vi "NIFPGA-MCS.ProcCases.vi"(0 "i ref in":refnum<vi>, 1 "selector":string, 2 "Data":T1, 3 "call cluster":T2={"Object"="", "Selector"="", "CallType"=enum."synchronous", "Async Object"="", "Async Selector"="", "Data Descriptor"="", "Data"=[], "Error #"=0, "Expire"=0}, 5 "error in (no error)":errorcluster) -> (14 "i ref out":refnum<vi>, 17 "answer cluster":T2={"Object"="", "Selector"="", "CallType"=enum."synchronous", "Async Object"="", "Async Selector"="", "Data Descriptor"="", "Data"=[], "Error #"=0, "Expire"=0}, 19 "error out":errorcluster)   [LabVIEW 2014, in "NIFPGA-MCS.lvlib"]
doc: "This method is called by a process from within the default case in the event loop. The methods of a class that are linked to events will be called from THIS method. Add your code here."
uses:
  NIFPGA-MCS.lvlib
  CSCore/CSSystem/CoreDefs/CoreDefs.call_type.ctl
  CSCore/BaseProcess/BaseProcess.descriptor string definition.ctl
  CSCore/CSSystem/CoreDefs/CoreDefs.rawDataType.ctl
  CSCore/CSSystem/CoreLib/CoreLib.string 2 byte array.vi
  CSCore/CSSystem/CoreLib/CoreLib.short 2 byte array.vi
  CSCore/CSSystem/CoreLib/CoreLib.int 2 byte array.vi
  CSCore/CSSystem/CoreLib/CoreLib.byte array 2 int.vi
  CSCore/CSSystem/CoreLib/CoreLib.double 2 byte array.vi
  CSCore/CSSystem/CoreLib/CoreLib.byte array 2 double.vi
  CSCore/CSSystem/CoreLib/CoreLib.lvlib
  CSCore/BaseProcess/BaseProcess.lvlib
  CSCore/CSApplicationBaseClasses/MCSBase/MCSBase.lvlib
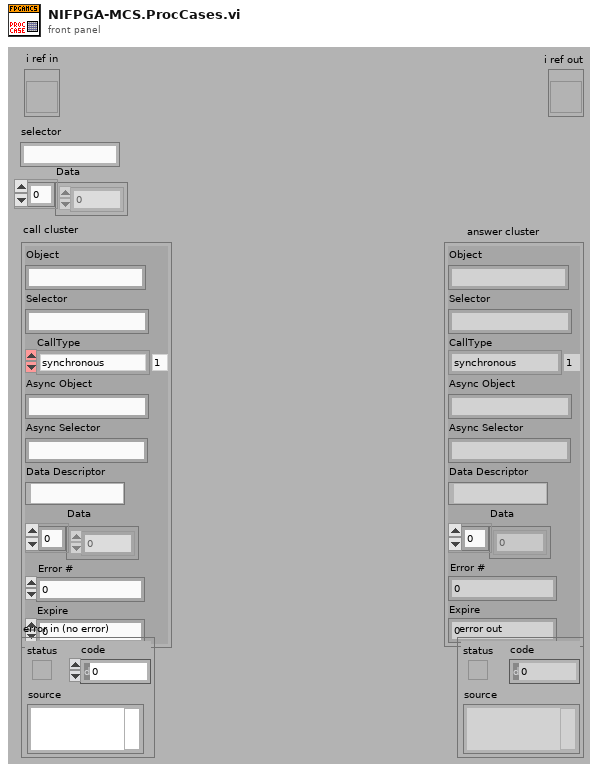
[diagram p1: front panel]
types:
  T1 = typedef "CoreDefs.rawDataType.ctl" = i8[]
  T2 = typedef "CoreDefs.call_type.ctl" = cluster{"Object":string, "Selector":string, "CallType":enum16{"simple", "synchronous", "asynchronous"}, "Async Object":string, "Async Selector":string, "Data Descriptor":T3, "Data":T1, "Error #":i32, "Expire":u32}
  T3 = typedef "BaseProcess.lvlib/BaseProcess.descriptor string definition.ctl" = string
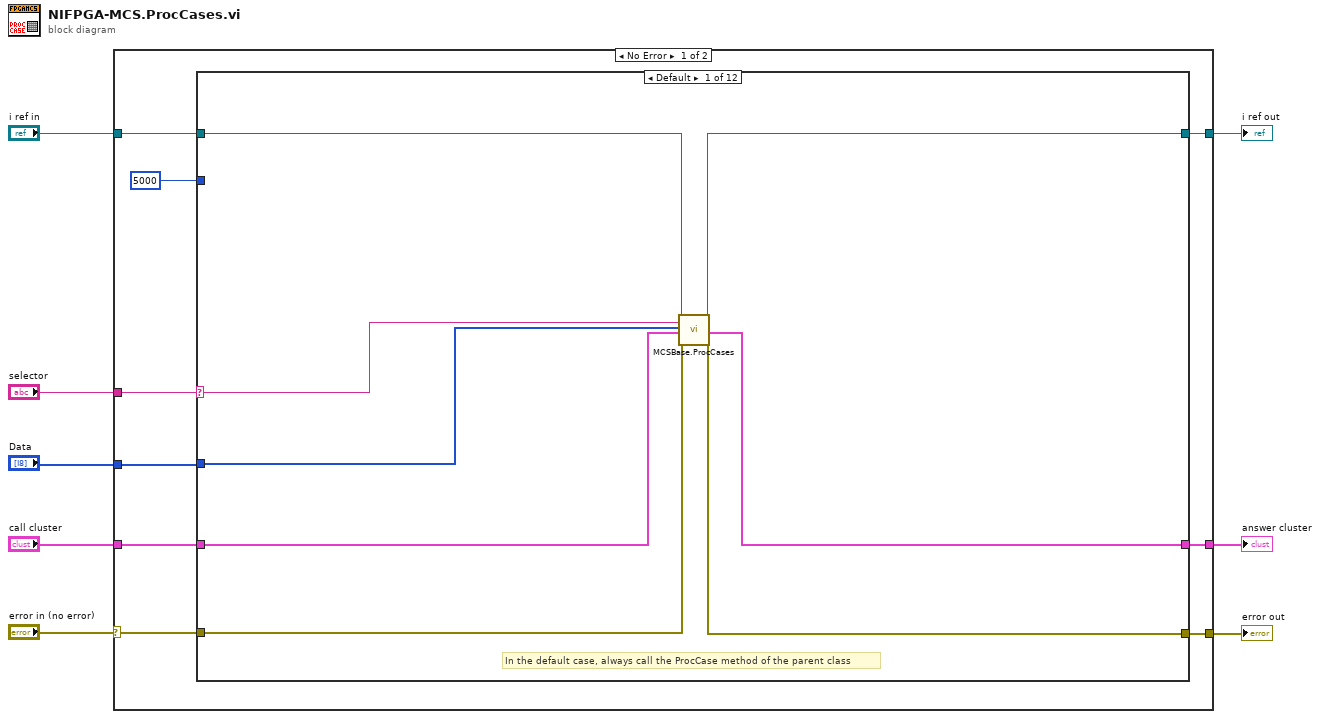
[diagram p0: block diagram]
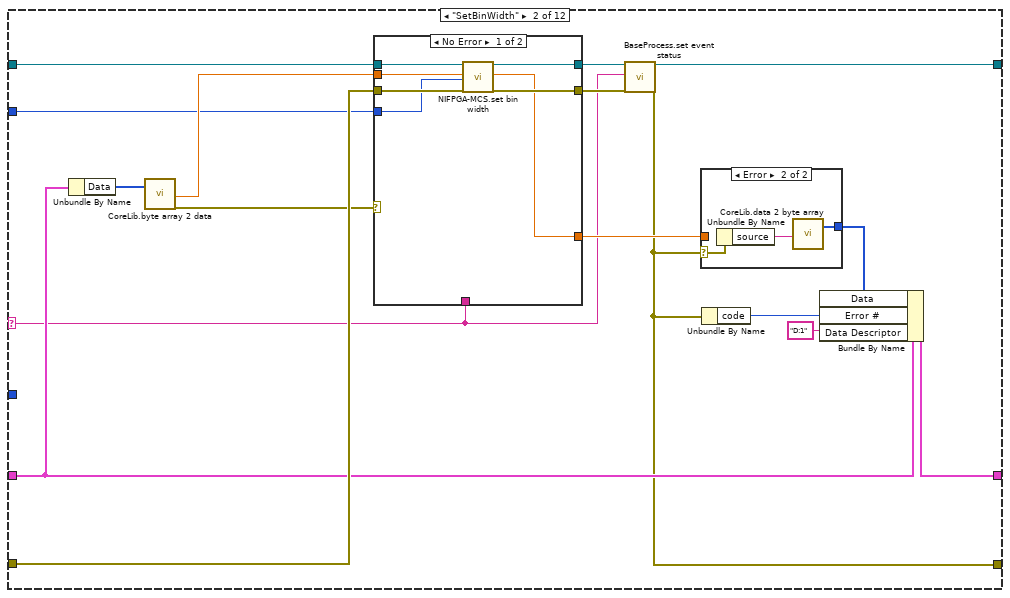
[diagram p2: hidden frame]
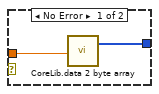
[diagram p3: hidden frame]
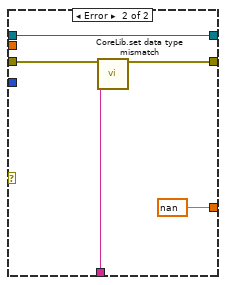
[diagram p4: hidden frame]
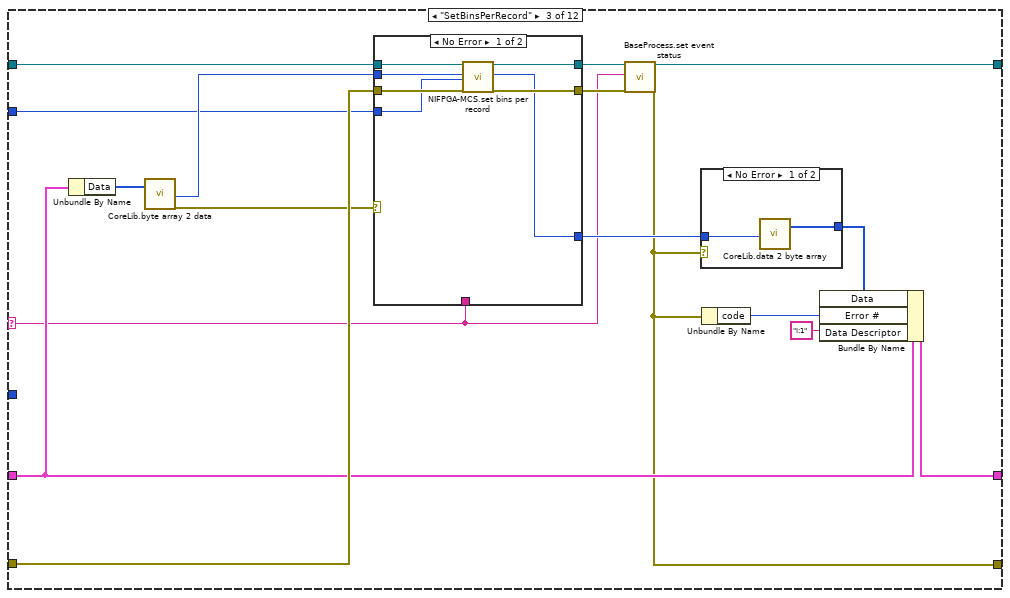
[diagram p5: hidden frame]
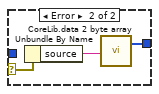
[diagram p6: hidden frame]
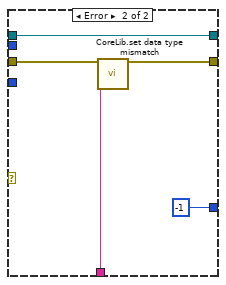
[diagram p7: hidden frame]
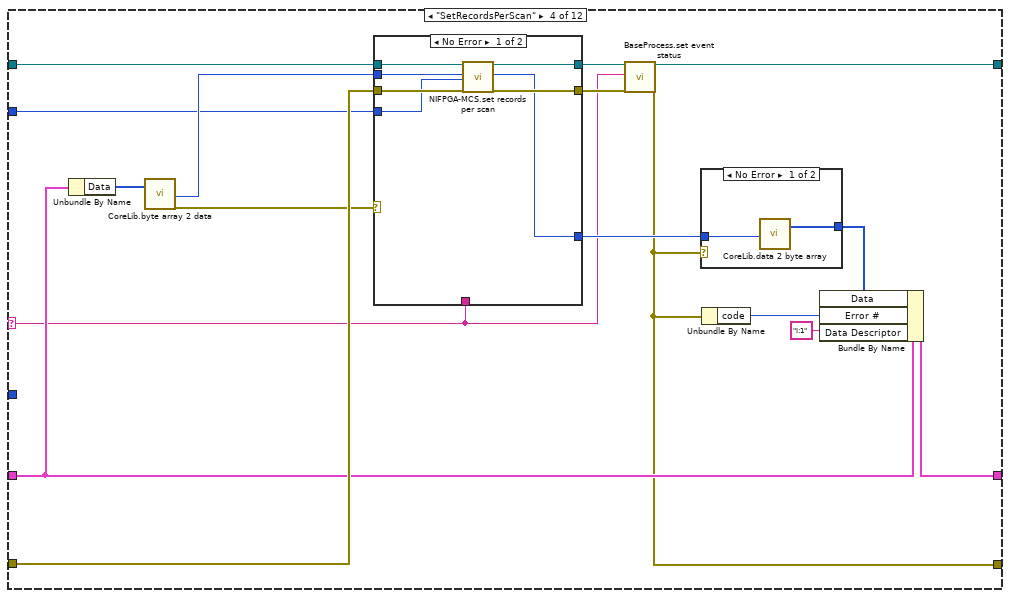
[diagram p8: hidden frame]
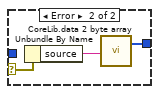
[diagram p9: hidden frame]
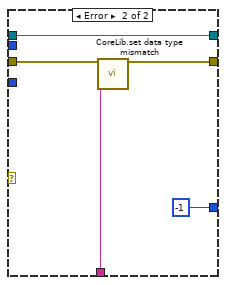
[diagram p10: hidden frame]
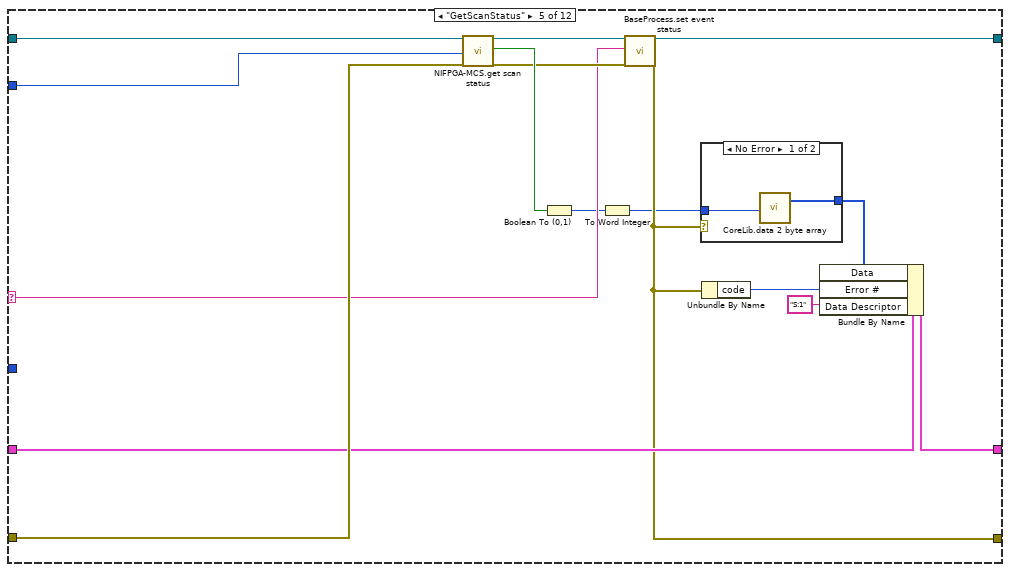
[diagram p11: hidden frame]
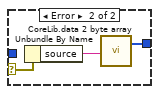
[diagram p12: hidden frame]
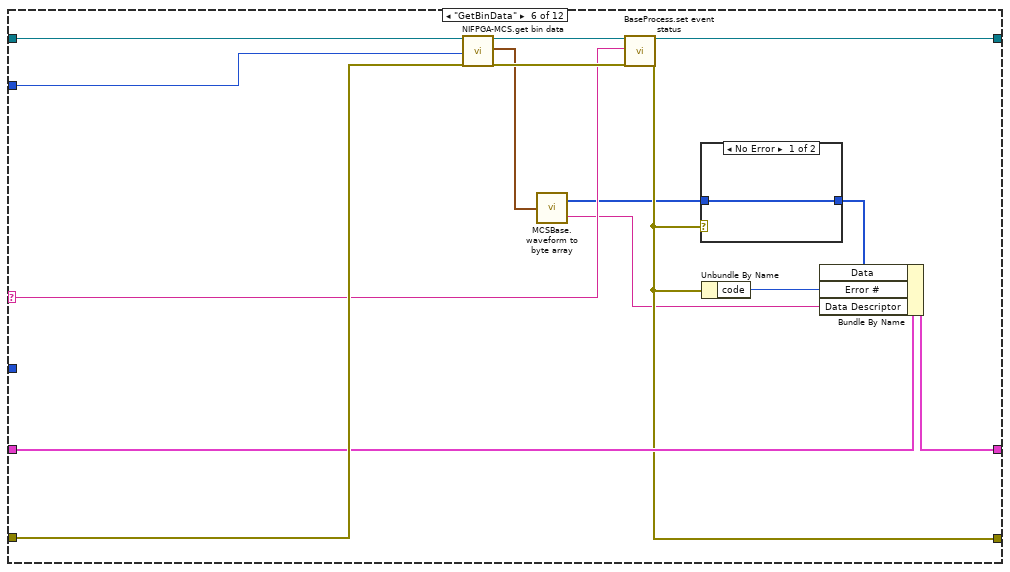
[diagram p13: hidden frame]
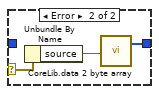
[diagram p14: hidden frame]
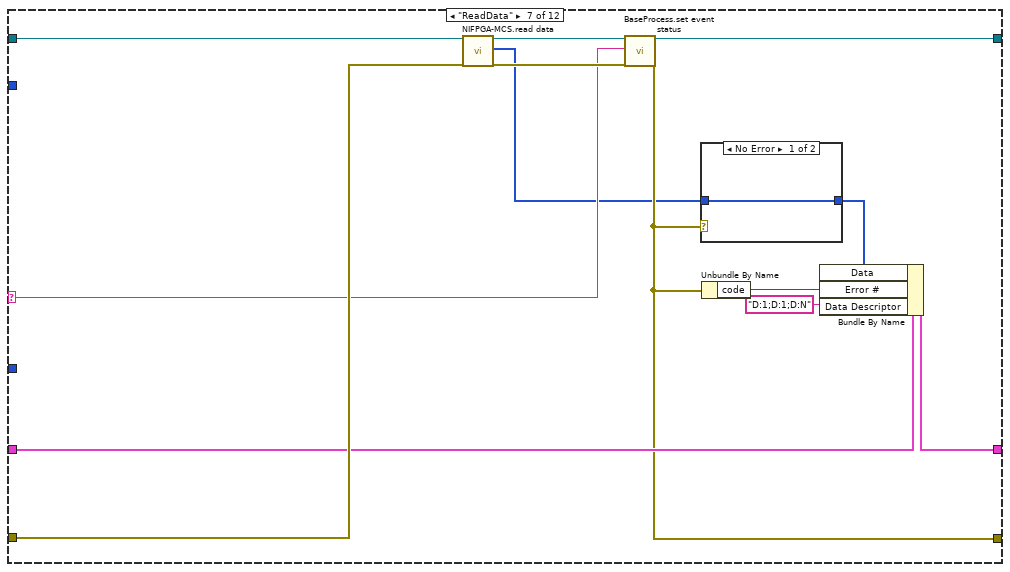
[diagram p15: hidden frame]
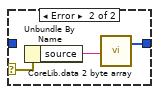
[diagram p16: hidden frame]
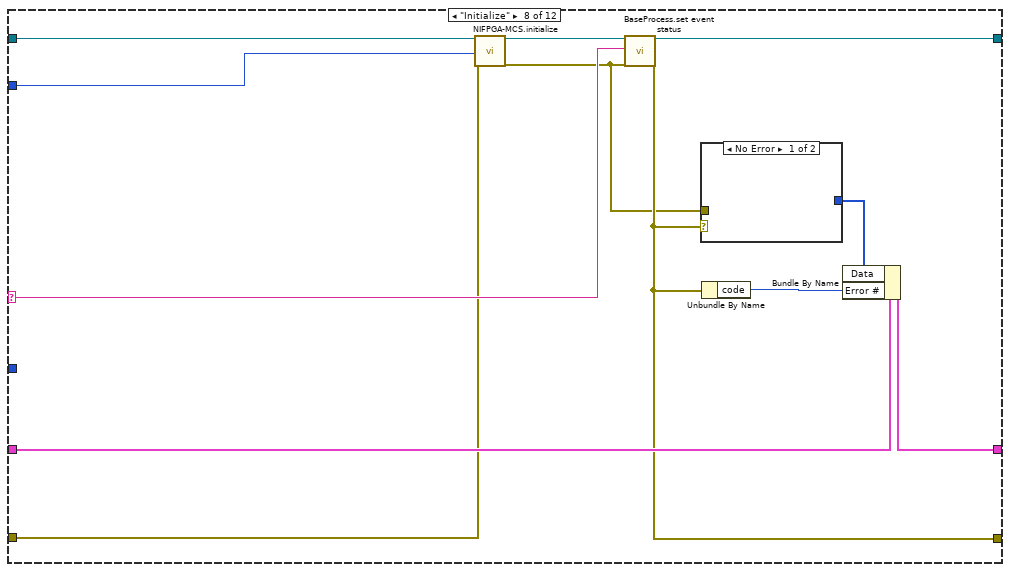
[diagram p17: hidden frame]
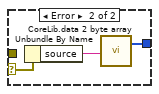
[diagram p18: hidden frame]
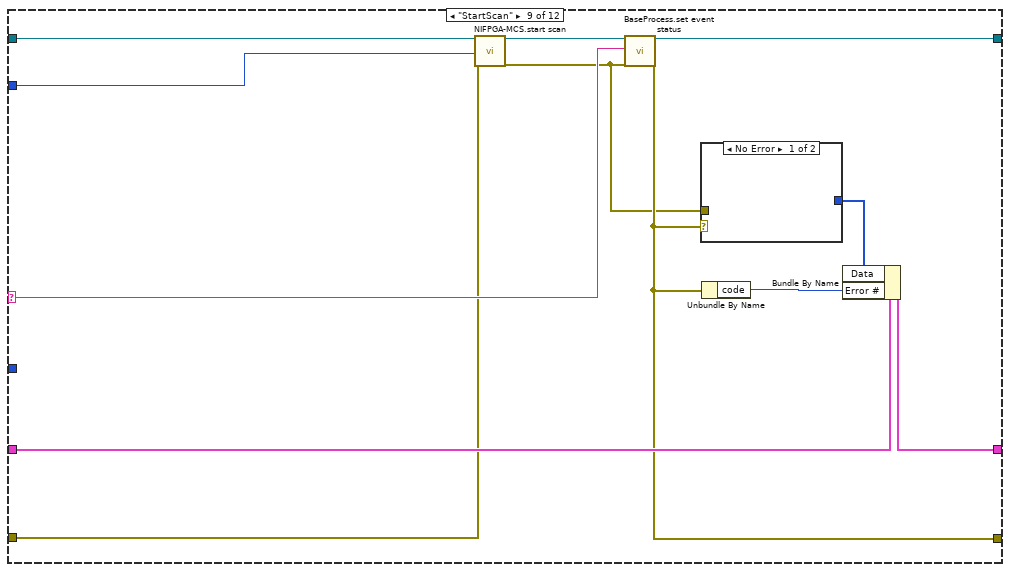
[diagram p19: hidden frame]
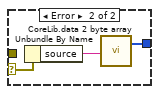
[diagram p20: hidden frame]
diagram:
  n1 = case shown="No Error" "error in (no error)" {
    selector: "error in (no error)" -> [w10 w259]
    tunnel: "selector" -> [w17 _]
    tunnel: [w16 w260] -> w7
    tunnel: "Data" -> [w15 _]
    tunnel: "call cluster" -> [w14 w260]
    tunnel: "i ref in" -> [w13 w261]
    tunnel: [w12 w261] -> w3
    tunnel: [w11 w259] -> w2
    frame No Error {
      n2 = case shown="Default" w17 {
        selector: w17 -> [w20 w32 w66 w100 w133 w154 w171 w191 w206 w221 w236 w250]
        tunnel: w15 -> [w18 _ _ _ _ _ _ _ _ _ _ _]
        tunnel: w13 -> [w19 w42 w76 w110 w143 w163 w180 w189 w204 w219 w234 w248]
        tunnel: [w25 w31 w65 w99 w132 w153 w170 w190 w205 w220 w235 w249] -> w12
        tunnel: w14 -> [w21 w38 w72 w106 w139 w160 w177 w195 w210 w225 w240 w254]
        tunnel: [w22 w37 w71 w105 w138 w159 w176 w194 w209 w224 w239 w253] -> w16
        tunnel: w10 -> [w24 w41 w75 w109 w142 w162 w179 w187 w202 w217 w232 w247]
        tunnel: [w23 w33 w67 w101 w134 w155 w172 w192 w207 w222 w237 w251] -> w11
        tunnel: 5000 -> [_ w26 w60 w94 w130 w152 _ w188 w203 w218 w233 _]
        frame Default {
          # "In the default case, always call the ProcCase method of the parent class"
          n3 = call "MCSBase.ProcCases.vi"("i ref in"=w19, "selector"=w20, "Data"=w18, "call cluster"=w21, "error in (no error)"=w24) -> ("i ref out"=w25:refnum<vi>, "answer cluster"=w22:T2, "error out"=w23:errorcluster)  [unwired: 12 in]
        }
        frame "SetBinWidth" {
          n4 = Unbundle By Name(w38) -> ("Data"=w29:T1)
          n5 = call-poly "CoreLib.byte array 2 data.vi"("byteArray"=w29) -> ("d64"=w28:dbl, "error out"=w27:errorcluster)  [unwired: 16 in, 1 out]
          n6 = case shown="No Error" w27 {
            tunnel: [w53 w59] -> w35
            tunnel: w42 -> [w54 w59]
            tunnel: w41 -> [w52 w58]
            tunnel: [w51 w57] -> w34
            tunnel: [w48 nan] -> w40
            tunnel: w32 -> [_ w55]
            tunnel: w28 -> [w50 _]
            tunnel: w26 -> [w49 _]
            frame No Error {
              n7 = call "NIFPGA-MCS.set bin width.vi"("i ref in"=w54, "binWidth [us]"=w50, "ms timeout (10000)"=w49, "error in (no error)"=w52) -> ("i ref out"=w53:refnum<vi>, "binWidth out [us]"=w48:dbl, "error out"=w51:errorcluster)  [unwired: 12 in, 1 out]
            }
            frame Error {
              n8 = call "CoreLib.set data type mismatch.vi"("error in (no error)"=w58, "error source"=w55) -> ("error out"=w57:errorcluster)  [unwired: 17 in]
            }
          }
          n9 = call "BaseProcess.set event status.vi"("i ref in"=w35, "EventStatus"=w32, "error in (no error)"=w34) -> ("i ref out"=w31:refnum<vi>, "error out"=w33:errorcluster)  [unwired: 14 in, 1 out]
          n10 = case shown="Error" w33 {
            selector: w33 -> [_ w47]
            tunnel: [w43 w46] -> w36
            tunnel: w40 -> [w44 _]
            frame No Error {
              n11 = call-poly "CoreLib.data 2 byte array.vi"("f64"=w44) -> ("byteArray out"=w43:T1)  [unwired: 18 in]
            }
            frame Error {
              n12 = Unbundle By Name(w47) -> ("source"=w45:string)
              n13 = call-poly "CoreLib.data 2 byte array.vi"("string"=w45) -> ("byteArray out"=w46:T1)  [unwired: 18 in]
            }
          }
          n14 = Unbundle By Name(w33) -> ("code"=w39:i32)
          n15 = Bundle By Name(cluster=w38, "Data"=w36, "Error #"=w39, "Data Descriptor"="D:1") -> (w37:T2)
        }
        frame "SetBinsPerRecord" {
          n16 = Unbundle By Name(w72) -> ("Data"=w63:T1)
          n17 = call-poly "CoreLib.byte array 2 data.vi"("byteArray"=w63) -> ("i32"=w62:i32, "error out"=w61:errorcluster)  [unwired: 16 in, 1 out]
          n18 = case shown="No Error" w61 {
            tunnel: [w87 w93] -> w69
            tunnel: w76 -> [w88 w93]
            tunnel: w75 -> [w86 w92]
            tunnel: [w85 w91] -> w68
            tunnel: [w82 -1] -> w74
            tunnel: w66 -> [_ w89]
            tunnel: w62 -> [w84 _]
            tunnel: w60 -> [w83 _]
            frame No Error {
              n19 = call "NIFPGA-MCS.set bins per record.vi"("i ref in"=w88, "binsPerRecord"=w84, "ms timeout (10000)"=w83, "error in (no error)"=w86) -> ("i ref out"=w87:refnum<vi>, "binsPerRecord out"=w82:i32, "error out"=w85:errorcluster)  [unwired: 12 in, 1 out]
            }
            frame Error {
              n20 = call "CoreLib.set data type mismatch.vi"("error in (no error)"=w92, "error source"=w89) -> ("error out"=w91:errorcluster)  [unwired: 17 in]
            }
          }
          n21 = call "BaseProcess.set event status.vi"("i ref in"=w69, "EventStatus"=w66, "error in (no error)"=w68) -> ("i ref out"=w65:refnum<vi>, "error out"=w67:errorcluster)  [unwired: 14 in, 1 out]
          n22 = case shown="No Error" w67 {
            selector: w67 -> [_ w81]
            tunnel: [w77 w80] -> w70
            tunnel: w74 -> [w78 _]
            frame No Error {
              n23 = call-poly "CoreLib.data 2 byte array.vi"("i32"=w78) -> ("byteArray out"=w77:T1)  [unwired: 18 in]
            }
            frame Error {
              n24 = Unbundle By Name(w81) -> ("source"=w79:string)
              n25 = call-poly "CoreLib.data 2 byte array.vi"("string"=w79) -> ("byteArray out"=w80:T1)  [unwired: 18 in]
            }
          }
          n26 = Unbundle By Name(w67) -> ("code"=w73:i32)
          n27 = Bundle By Name(cluster=w72, "Data"=w70, "Error #"=w73, "Data Descriptor"="I:1") -> (w71:T2)
        }
        frame "SetRecordsPerScan" {
          n28 = Unbundle By Name(w106) -> ("Data"=w97:T1)
          n29 = call-poly "CoreLib.byte array 2 data.vi"("byteArray"=w97) -> ("i32"=w96:i32, "error out"=w95:errorcluster)  [unwired: 16 in, 1 out]
          n30 = case shown="No Error" w95 {
            tunnel: [w121 w127] -> w103
            tunnel: w110 -> [w122 w127]
            tunnel: w109 -> [w120 w126]
            tunnel: [w119 w125] -> w102
            tunnel: [w116 -1] -> w108
            tunnel: w100 -> [_ w123]
            tunnel: w96 -> [w118 _]
            tunnel: w94 -> [w117 _]
            frame No Error {
              n31 = call "NIFPGA-MCS.set records per scan.vi"("i ref in"=w122, "recordsPerScan"=w118, "ms timeout (10000)"=w117, "error in (no error)"=w120) -> ("i ref out"=w121:refnum<vi>, "recordsPerScan out"=w116:i32, "error out"=w119:errorcluster)  [unwired: 12 in, 1 out]
            }
            frame Error {
              n32 = call "CoreLib.set data type mismatch.vi"("error in (no error)"=w126, "error source"=w123) -> ("error out"=w125:errorcluster)  [unwired: 17 in]
            }
          }
          n33 = call "BaseProcess.set event status.vi"("i ref in"=w103, "EventStatus"=w100, "error in (no error)"=w102) -> ("i ref out"=w99:refnum<vi>, "error out"=w101:errorcluster)  [unwired: 14 in, 1 out]
          n34 = case shown="No Error" w101 {
            selector: w101 -> [_ w115]
            tunnel: [w111 w114] -> w104
            tunnel: w108 -> [w112 _]
            frame No Error {
              n35 = call-poly "CoreLib.data 2 byte array.vi"("i32"=w112) -> ("byteArray out"=w111:T1)  [unwired: 18 in]
            }
            frame Error {
              n36 = Unbundle By Name(w115) -> ("source"=w113:string)
              n37 = call-poly "CoreLib.data 2 byte array.vi"("string"=w113) -> ("byteArray out"=w114:T1)  [unwired: 18 in]
            }
          }
          n38 = Unbundle By Name(w101) -> ("code"=w107:i32)
          n39 = Bundle By Name(cluster=w106, "Data"=w104, "Error #"=w107, "Data Descriptor"="I:1") -> (w105:T2)
        }
        frame "GetScanStatus" {
          n40 = call "NIFPGA-MCS.get scan status.vi"("i ref in"=w143, "ms timeout (10000)"=w130, "error in (no error)"=w142) -> ("i ref out"=w136:refnum<vi>, "scanFinished ?"=w141:bool, "error out"=w135:errorcluster)  [unwired: 13 in, 1 out]
          n41 = Boolean To (0,1)(Boolean=w141) -> (0, 1=w129:i16)
          n42 = To Word Integer(number=w129) -> (16bit integer=w128:i16)
          n43 = call "BaseProcess.set event status.vi"("i ref in"=w136, "EventStatus"=w133, "error in (no error)"=w135) -> ("i ref out"=w132:refnum<vi>, "error out"=w134:errorcluster)  [unwired: 14 in, 1 out]
          n44 = case shown="No Error" w134 {
            selector: w134 -> [_ w148]
            tunnel: [w144 w147] -> w137
            tunnel: w128 -> [w145 _]
            frame No Error {
              n45 = call-poly "CoreLib.data 2 byte array.vi"("i16"=w145) -> ("byteArray out"=w144:T1)  [unwired: 18 in]
            }
            frame Error {
              n46 = Unbundle By Name(w148) -> ("source"=w146:string)
              n47 = call-poly "CoreLib.data 2 byte array.vi"("string"=w146) -> ("byteArray out"=w147:T1)  [unwired: 18 in]
            }
          }
          n48 = Unbundle By Name(w134) -> ("code"=w140:i32)
          n49 = Bundle By Name(cluster=w139, "Data"=w137, "Error #"=w140, "Data Descriptor"="S:1") -> (w138:T2)
        }
        frame "GetBinData" {
          n50 = call "NIFPGA-MCS.get bin data.vi"("i ref in"=w163, "ms timeout (10000)"=w152, "error in (no error)"=w162) -> ("i ref out"=w157:refnum<vi>, "Output Waveform"=w151:waveform(dbl), "error out"=w156:errorcluster)  [unwired: 14 in]
          n51 = call "MCSBase.waveform to byte array.vi"("Waveform"=w151) -> ("byteArray out"=w150:T1, "dataDescriptor"=w149:string)
          n52 = call "BaseProcess.set event status.vi"("i ref in"=w157, "EventStatus"=w154, "error in (no error)"=w156) -> ("i ref out"=w153:refnum<vi>, "error out"=w155:errorcluster)  [unwired: 14 in, 1 out]
          n53 = case shown="No Error" w155 {
            selector: w155 -> [_ w167]
            tunnel: [w164 w166] -> w158
            tunnel: w150 -> [w164 _]
            frame No Error {
            }
            frame Error {
              n54 = Unbundle By Name(w167) -> ("source"=w165:string)
              n55 = call-poly "CoreLib.data 2 byte array.vi"("string"=w165) -> ("byteArray out"=w166:T1)  [unwired: 18 in]
            }
          }
          n56 = Unbundle By Name(w155) -> ("code"=w161:i32)
          n57 = Bundle By Name(cluster=w160, "Data"=w158, "Error #"=w161, "Data Descriptor"=w149) -> (w159:T2)
        }
        frame "ReadData" {
          n58 = call "NIFPGA-MCS.read data.vi"("i ref in"=w180, "error in (no error)"=w179) -> ("i ref out"=w174:refnum<vi>, "Output Waveform"=w169:T1, "error out"=w173:errorcluster)  [unwired: 15 in]
          n59 = call "BaseProcess.set event status.vi"("i ref in"=w174, "EventStatus"=w171, "error in (no error)"=w173) -> ("i ref out"=w170:refnum<vi>, "error out"=w172:errorcluster)  [unwired: 14 in, 1 out]
          n60 = case shown="No Error" w172 {
            selector: w172 -> [_ w184]
            tunnel: [w181 w183] -> w175
            tunnel: w169 -> [w181 _]
            frame No Error {
            }
            frame Error {
              n61 = Unbundle By Name(w184) -> ("source"=w182:string)
              n62 = call-poly "CoreLib.data 2 byte array.vi"("string"=w182) -> ("byteArray out"=w183:T1)  [unwired: 18 in]
            }
          }
          n63 = Unbundle By Name(w172) -> ("code"=w178:i32)
          n64 = Bundle By Name(cluster=w177, "Data"=w175, "Error #"=w178, "Data Descriptor"=T3 "D:1;D:1;D:N") -> (w176:T2)
        }
        frame "Initialize" {
          n65 = call "NIFPGA-MCS.initialize.vi"("i ref in"=w189, "ms timeout (10000)"=w188, "error in (no error)"=w187) -> ("i ref out"=w186:refnum<vi>, "error out"=w185:errorcluster)  [unwired: 14 in, 1 out]
          n66 = call "BaseProcess.set event status.vi"("i ref in"=w186, "EventStatus"=w191, "error in (no error)"=w185) -> ("i ref out"=w190:refnum<vi>, "error out"=w192:errorcluster)  [unwired: 14 in, 1 out]
          n67 = case shown="No Error" w192 {
            selector: w192 -> [_ w199]
            tunnel: [_ w198] -> w193
            tunnel: w185 -> [_ _]
            frame No Error {
            }
            frame Error {
              n68 = Unbundle By Name(w199) -> ("source"=w197:string)
              n69 = call-poly "CoreLib.data 2 byte array.vi"("string"=w197) -> ("byteArray out"=w198:T1)  [unwired: 18 in]
            }
          }
          n70 = Unbundle By Name(w192) -> ("code"=w196:i32)
          n71 = Bundle By Name(cluster=w195, "Data"=w193, "Error #"=w196) -> (w194:T2)
        }
        frame "StartScan" {
          n72 = call "NIFPGA-MCS.start scan.vi"("i ref in"=w204, "ms timeout (10000)"=w203, "error in (no error)"=w202) -> ("i ref out"=w201:refnum<vi>, "error out"=w200:errorcluster)  [unwired: 14 in, 1 out]
          n73 = call "BaseProcess.set event status.vi"("i ref in"=w201, "EventStatus"=w206, "error in (no error)"=w200) -> ("i ref out"=w205:refnum<vi>, "error out"=w207:errorcluster)  [unwired: 14 in, 1 out]
          n74 = case shown="No Error" w207 {
            selector: w207 -> [_ w214]
            tunnel: [_ w213] -> w208
            tunnel: w200 -> [_ _]
            frame No Error {
            }
            frame Error {
              n75 = Unbundle By Name(w214) -> ("source"=w212:string)
              n76 = call-poly "CoreLib.data 2 byte array.vi"("string"=w212) -> ("byteArray out"=w213:T1)  [unwired: 18 in]
            }
          }
          n77 = Unbundle By Name(w207) -> ("code"=w211:i32)
          n78 = Bundle By Name(cluster=w210, "Data"=w208, "Error #"=w211) -> (w209:T2)
        }
        frame "StopScan" {
          n79 = call "NIFPGA-MCS.stop scan.vi"("i ref in"=w219, "ms timeout (10000)"=w218, "error in (no error)"=w217) -> ("i ref out"=w216:refnum<vi>, "error out"=w215:errorcluster)  [unwired: 14 in, 1 out]
          n80 = call "BaseProcess.set event status.vi"("i ref in"=w216, "EventStatus"=w221, "error in (no error)"=w215) -> ("i ref out"=w220:refnum<vi>, "error out"=w222:errorcluster)  [unwired: 14 in, 1 out]
          n81 = case shown="No Error" w222 {
            selector: w222 -> [_ w229]
            tunnel: [_ w228] -> w223
            tunnel: w215 -> [_ _]
            frame No Error {
            }
            frame Error {
              n82 = Unbundle By Name(w229) -> ("source"=w227:string)
              n83 = call-poly "CoreLib.data 2 byte array.vi"("string"=w227) -> ("byteArray out"=w228:T1)  [unwired: 18 in]
            }
          }
          n84 = Unbundle By Name(w222) -> ("code"=w226:i32)
          n85 = Bundle By Name(cluster=w225, "Data"=w223, "Error #"=w226) -> (w224:T2)
        }
        frame "Close" {
          n86 = call "NIFPGA-MCS.close.vi"("i ref in"=w234, "ms timeout (10000)"=w233, "error in (no error)"=w232) -> ("i ref out"=w231:refnum<vi>, "error out"=w230:errorcluster)  [unwired: 14 in, 1 out]
          n87 = call "BaseProcess.set event status.vi"("i ref in"=w231, "EventStatus"=w236, "error in (no error)"=w230) -> ("i ref out"=w235:refnum<vi>, "error out"=w237:errorcluster)  [unwired: 14 in, 1 out]
          n88 = case shown="No Error" w237 {
            selector: w237 -> [_ w244]
            tunnel: [_ w243] -> w238
            tunnel: w230 -> [_ _]
            frame No Error {
            }
            frame Error {
              n89 = Unbundle By Name(w244) -> ("source"=w242:string)
              n90 = call-poly "CoreLib.data 2 byte array.vi"("string"=w242) -> ("byteArray out"=w243:T1)  [unwired: 18 in]
            }
          }
          n91 = Unbundle By Name(w237) -> ("code"=w241:i32)
          n92 = Bundle By Name(cluster=w240, "Data"=w238, "Error #"=w241) -> (w239:T2)
        }
        frame "Reset" {
          n93 = call "NIFPGA-MCS.reset.vi"("i ref in"=w248, "error in (no error)"=w247) -> ("i ref out"=w246:refnum<vi>, "error out"=w245:errorcluster)  [unwired: 16 in]
          n94 = call "BaseProcess.set event status.vi"("i ref in"=w246, "EventStatus"=w250, "error in (no error)"=w245) -> ("i ref out"=w249:refnum<vi>, "error out"=w251:errorcluster)  [unwired: 14 in, 1 out]
          n95 = case shown="No Error" w251 {
            selector: w251 -> [_ w258]
            tunnel: [_ w257] -> w252
            tunnel: w245 -> [_ _]
            frame No Error {
            }
            frame Error {
              n96 = Unbundle By Name(w258) -> ("source"=w256:string)
              n97 = call-poly "CoreLib.data 2 byte array.vi"("string"=w256) -> ("byteArray out"=w257:T1)  [unwired: 18 in]
            }
          }
          n98 = Unbundle By Name(w251) -> ("code"=w255:i32)
          n99 = Bundle By Name(cluster=w254, "Data"=w252, "Error #"=w255) -> (w253:T2)
        }
      }
    }
    frame Error {
    }
  }
  "answer cluster" <- w7
  "i ref out" <- w3
  "error out" <- w2
